vi "Example Threshold - Power Callback.vi"(4 "Power":refnum<user-event>, 5 "Event Data":cluster{"sender":refnum<k24>, "power":i32}, 6 "Control Ref":refnum<k24>, 7 "Event Common Data":T1) -> ()   [LabVIEW 2013]
uses:
  C:/tf/play/labview/Tinkerforge.dll
  Tinkerforge.dll
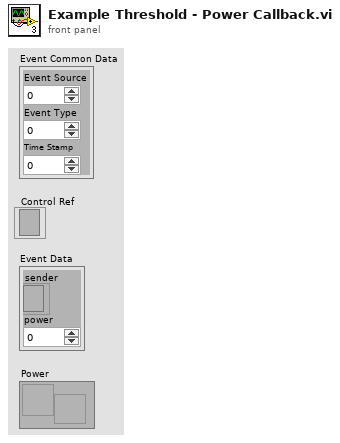
[diagram p1: front panel]
types:
  T1 = cluster{"Event Source":i32, "Event Type":u32, "Time Stamp":u32}
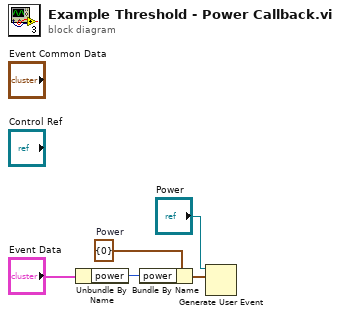
[diagram p0: block diagram]
diagram:
  w4 = cluster{"power":i32} {"power"=0}  # Power
  n1 = Unbundle By Name("Event Data") -> ("power"=w3:i32)
  n2 = Bundle By Name(cluster=w4, "power"=w3) -> (w2:cluster{"power":i32})
  n3 = Generate User Event(user event="Power", event data cluster=w2) -> ()  [unwired: 2 in, 2 out]
